vi "REF Array Add or Remove.vi"(8 "error in (no error)":errorcluster, 11 "REF Channels in":T1=[{"Enable?"=FALSE, "Channel"=13, "Frequency"=0.1, "Phase"=0.0, "TC"=1e-05, "Roll-Off"=1}] {"Roll-Off" min=1 max=4; "TC" min=1e-06 max=100.0 format="%#_3p"; "Phase" format="%#_3p"; "Frequency" min=1e-06 max=102400.0 format="%#_6p"; "Channel" min=1}) -> (0 "error out":errorcluster, 3 "REF Channels out":T1=[{"Enable?"=FALSE, "Channel"=13, "Frequency"=0.1, "Phase"=0.0, "TC"=1e-05, "Roll-Off"=1}] {"Roll-Off" min=1 max=4; "TC" min=1e-06 max=100.0 format="%#_3p"; "Phase" format="%#_3p"; "Frequency" min=1e-06 max=102400.0 format="%#_6p"; "Channel" min=1})   [LabVIEW 2019, in "Instrument.Lockin.lvlib" / "Instrument.DAQ.lvclass"]
uses:
  Instrument.DAQ.lvclass
  Typedefs/REF.Channel--Cluster--Array.ctl
  Typedefs/REF.Channel--Cluster.ctl
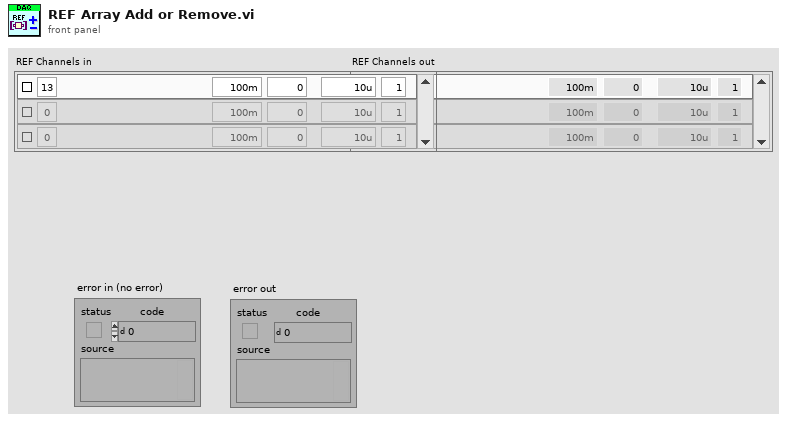
[diagram p1: front panel]
types:
  T1 = typedef "Instrument.Lockin.lvlib/Instrument.DAQ.lvclass/REF.Channel--Cluster--Array.ctl" = T2[]
  T2 = typedef "Instrument.Lockin.lvlib/Instrument.DAQ.lvclass/REF.Channel--Cluster.ctl" = cluster{"Enable?":bool, "Channel":i32, "Frequency":dbl, "Phase":dbl, "TC":dbl, "Roll-Off":i32}
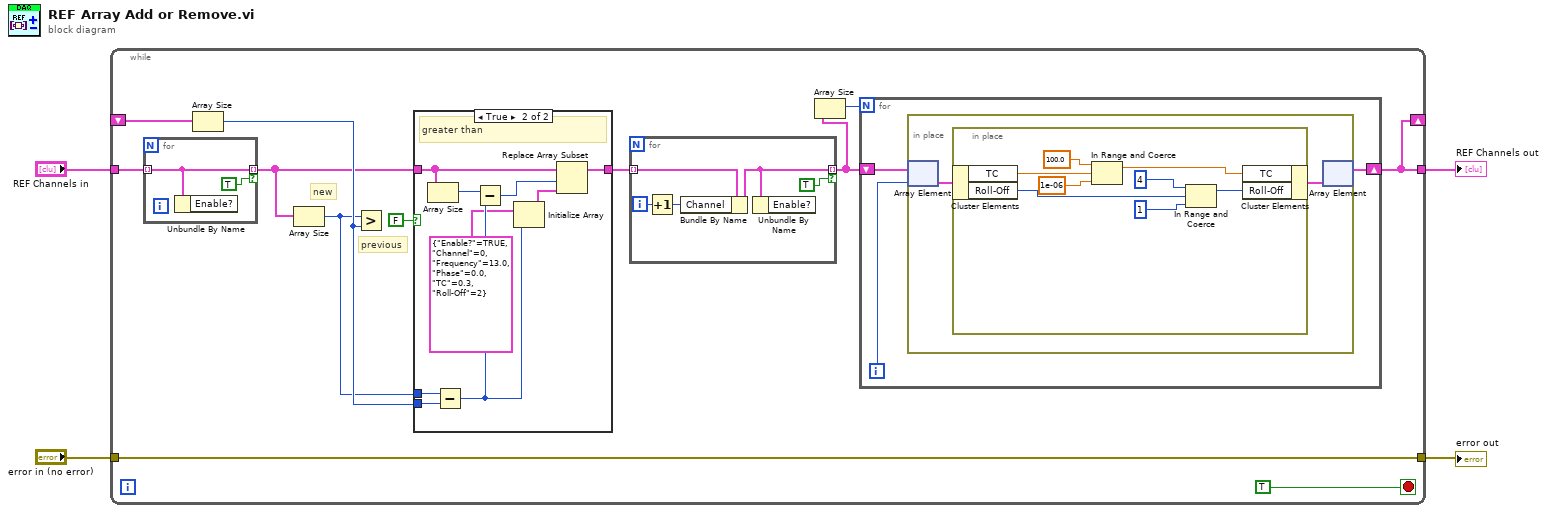
[diagram p0: block diagram]
diagram:
  n1 = while {
    tunnel: "REF Channels in" -> [w7]
    tunnel: [w10] -> w3
    tunnel: "error in (no error)" -> [w15]
    tunnel: [w15] -> w1
    shift-right: [w10] -> _
    shift-left: _ -> [w13]
    stop <- TRUE stop-if-true
    # "new"
    # "previous"
    n2 = for {
      tunnel: w7 -> [w36] mode=indexing
      tunnel: [w36] -> w6 mode=indexing if=TRUE
      n3 = Unbundle By Name(w36) -> ()  [unwired: 1 out]
    }
    n4 = Array Size(array=w13) -> (size(s)=w12:i32)
    n5 = Array Size(array=w6) -> (size(s)=w11:i32)
    n6 = Greater?(x=w11, y=w12) -> ()  [unwired: 1 out]
    n7 = case shown="True" FALSE {
      tunnel: w6 -> [w37 w42]
      tunnel: w11 -> [_ w46]
      tunnel: [w37 w43] -> w16
      tunnel: w12 -> [_ w45]
      frame False {
        # "less than or equal"
      }
      frame True {
        # "greater than"
        n8 = Array Size(array=w42) -> (size(s)=w41:i32)
        n9 = Subtract(x=w46, y=w45) -> (x-y=w40:i32)
        n10 = Subtract(x=w41, y=w40) -> (x-y=w39:i32)
        n11 = Initialize Array(T2 {"Enable?"=TRUE, "Channel"=0, "Frequency"=13.0, "Phase"=0.0, "TC"=0.3, "Roll-Off"=2} ("REF"), w40) -> (w44:T2[])
        n12 = Replace Array Subset(array=w42, new element=w44, index=w39) -> (w43:T2[])
      }
    }
    n13 = for {
      tunnel: w16 -> [w32] mode=indexing
      tunnel: [w31] -> w8 mode=indexing if=TRUE
      i -> [w33]
      n14 = Increment(x=w33) -> (x+1=w34:i32)
      n15 = Bundle By Name(cluster=w32, "Channel"=w34) -> (w31:T2)
      n16 = Unbundle By Name(w31) -> ()  [unwired: 1 out]
    }
    n17 = Array Size(array=w8) -> (size(s)=w9:i32)
    n18 = for {
      N: w9 -> [_]
      shift-right: [w18] -> w10
      shift-left: w8 -> [w19]
      i -> [w17]
      n19 = in-place {
        n20 = in-place-array #1(w19, w17) -> (w21:T2)
        n21 = in-place {
          n22 = in-place-cluster #2(w21) -> ("TC"=w25:dbl, "Roll-Off"=w24:i32)
          n23 = In Range and Coerce(upper limit=100.0, x=w25, lower limit=1e-06) -> (coerced(x)=w22:dbl)  [unwired: 1 out]
          n24 = In Range and Coerce(upper limit=4, x=w24, lower limit=1) -> (coerced(x)=w23:i32)  [unwired: 1 out]
          n25 = in-place-cluster #2("TC"=w22, "Roll-Off"=w23) -> (w20:T2)
        }
        n26 = in-place-array #1(w20) -> (w18:T2[])  [unwired: 1 out]
      }
    }
  }
  "REF Channels out" <- w3
  "error out" <- w1
